vi "ControlShutter.vi"() -> ()   [LabVIEW 2021]
panel:
  out "error out":errorcluster
  in  "stop":bool
  in  "Deg":u16
  in  "VISA Refnum in":refnum<visa-resource-name>
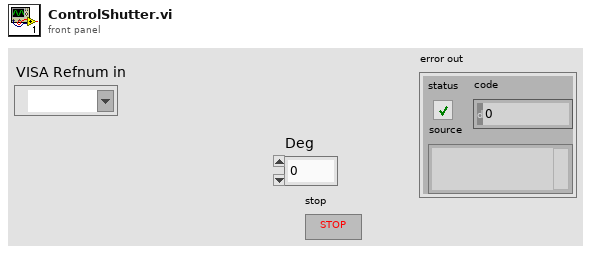
[diagram p1: front panel]
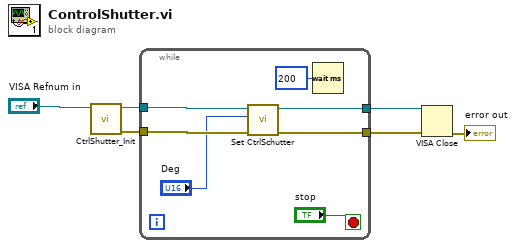
[diagram p0: block diagram]
diagram:
  n1 = call "CtrlShutter_Init.vi"("VISA Refnum in"="VISA Refnum in") -> ("error out"=w5:errorcluster, "VISA Refnum out"=w6:refnum<visa-resource-name>)  [unwired: 8 in, 1 out]
  n2 = while {
    tunnel: w6 -> [w13]
    tunnel: w5 -> [w12]
    tunnel: [w8] -> w3
    tunnel: [w7] -> w2
    stop <- "stop" stop-if-true
    n3 = call "Set CtrlSchutter.vi"("VISA Refnum in"=w13, "Deg"="Deg", "error in (no error)"=w12) -> ("VISA Refnum out"=w8:refnum<visa-resource-name>, "error out"=w7:errorcluster)  [unwired: 5 in, 1 out]
    n4 = Wait (ms)(milliseconds to wait=u32 200) -> ()  [unwired: 1 out]
  }
  n5 = VISA Close(VISA resource name=w3, error in (no error)=w2) -> (error out=→"error out":errorcluster)
